vi "GoToTest.vi"(8 "command\nenum":T1, 9 "Robot In":T2={"id"=0, "function"=enum."Attacker", "x"=0.0, "y"=0.0, "orientation"=0.0, "v_tangent"=0.0, "v_normal"=0.0, "v_ang"=0.0, "kick_x"=0.0, "kick_z"=0.0, "dribble"=FALSE, "Timestamp"=timestamp(0 s since 1904-01-01), "dest_x"=0.0, "dest_y"=0.0, "dest_orientation"=0.0, "estimatives"={"est_v_tangent"=0.0, "est_v_normal"=0.0, "est_vx"=0.0, "est_vy"=0.0, "Pos Robot Est"=[]}, "dest_x_kick"=0.0, "dest_y_kick"=0.0, "Gap Coord"=[], "States"=enum."GoToTangent"}, 10 "Ball":dbl[](array[numeric])=[-1986.6092529296875, -3009.6396484375], 11 "GoTo point":dbl[](array[numeric])=[0.0, 0.0, 0.0]) -> (1 "Robot Out":T2={"id"=0, "function"=enum."Attacker", "x"=0.0, "y"=0.0, "orientation"=0.0, "v_tangent"=0.0, "v_normal"=0.0, "v_ang"=0.0, "kick_x"=0.0, "kick_z"=0.0, "dribble"=FALSE, "Timestamp"=timestamp(0 s since 1904-01-01), "dest_x"=0.0, "dest_y"=0.0, "dest_orientation"=0.0, "estimatives"={"est_v_tangent"=0.0, "est_v_normal"=0.0, "est_vx"=0.0, "est_vy"=0.0, "Pos Robot Est"=[]}, "dest_x_kick"=0.0, "dest_y_kick"=0.0, "Gap Coord"=[], "States"=enum."GoToTangent"})   [LabVIEW 2016]
uses:
  Core/AI Robot.ctl
  Intel/Functions Enum.ctl
  Intel/AttackerStates.ctl
  Intel/Command Enum.ctl
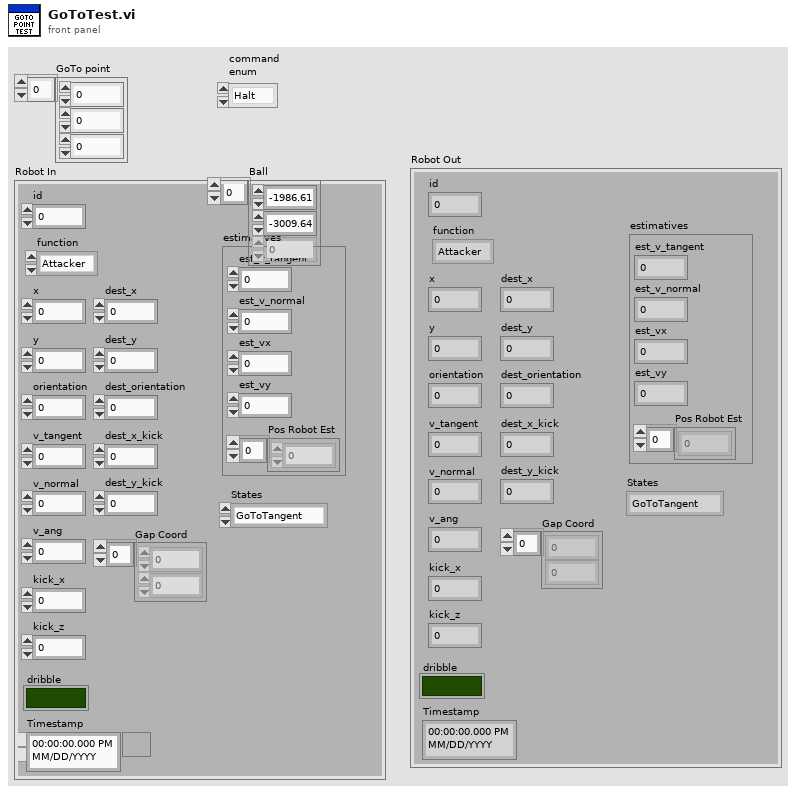
[diagram p1: front panel]
types:
  T1 = typedef "Command Enum.ctl" = enum16{"Halt", "Stop", "Force Start", "PKA Normal Start", "Prepare Kickoff Ally", "PKE Normal Start", "Prepare Kickoff Enemy", "Prepare Penalty Ally", "PPA Normal Start", "Prepare Penalty Enemy", "PPE Normal Start", "Direct Free Enemy", "Direct Free Ally", "Indirect Free Enemy", "Indirect Free Ally", "Timeout Enemy", "Timeout Ally", "Goal Enemy", "Goal Ally", "Ball Placement Enemy", "Ball Placement Ally", "Normal Half Time", "Extra Time Break", "Extra Half Time", "None", "Post Game"}
  T2 = typedef "AI Robot.ctl" = cluster{"id":u32, "function":T3, "x":dbl, "y":dbl, "orientation":dbl, "v_tangent":dbl, "v_normal":dbl, "v_ang":dbl, "kick_x":dbl, "kick_z":dbl, "dribble":bool, "Timestamp":timestamp, "dest_x":dbl, "dest_y":dbl, "dest_orientation":dbl, "estimatives":cluster{"est_v_tangent":dbl, "est_v_normal":dbl, "est_vx":dbl, "est_vy":dbl, "Pos Robot Est":dbl[]}, "dest_x_kick":dbl, "dest_y_kick":dbl, "Gap Coord":dbl[], "States":T4}
  T3 = typedef "Functions Enum.ctl" = enum16{"Attacker", "Goalie", "Defender", "Striker", "Goto 0", "Dummy", "Kicker", "ZigZag"}
  T4 = typedef "AttackerStates.ctl" = enum16{"Pass", "GoToTangent", "BallGetting", "GoToKick", ""}
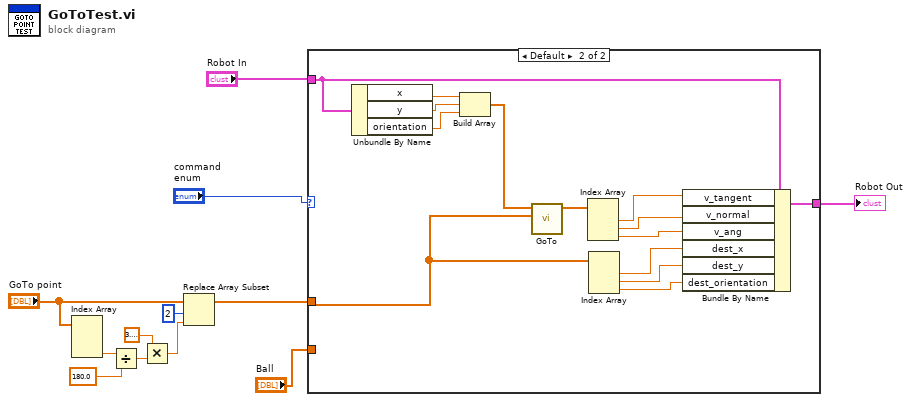
[diagram p0: block diagram]
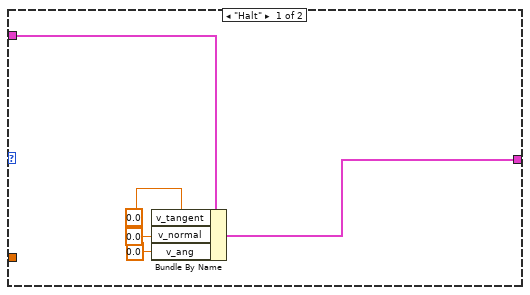
[diagram p2: hidden frame]
diagram:
  n1 = Index Array(array="GoTo point") -> (element #3=w6:dbl)  [unwired: 3 in, 2 out]
  n2 = Divide(x=w6, y=180.0) -> (x/y=w4:dbl)
  n3 = Multiply(x=3.141592653589793, y=w4) -> (x*y=w3:dbl)
  n4 = Replace Array Subset(array="GoTo point", new element=w3, index=2) -> (w7:dbl[])
  n5 = case shown="Default" "command\nenum" {
    tunnel: [w13 w22] -> w11
    tunnel: "Robot In" -> [w17 w27]
    tunnel: w7 -> [_ w19]
    tunnel: "Ball" -> [_ _]
    frame "Halt" {
      n6 = Bundle By Name(cluster=w17, "v_tangent"=0.0, "v_normal"=0.0, "v_ang"=0.0) -> (w13:T2)
    }
    frame Default {
      n7 = Unbundle By Name(w27) -> ("x"=w31:dbl, "y"=w30:dbl, "orientation"=w29:dbl)
      n8 = Build Array(w31, w30, w29) -> (w28:dbl[])
      n9 = call "GoTo.vi"("Target"=w19, "Position"=w28) -> ("Output\nVelocity"=w26:dbl[])  [unwired: 8 in, 1 out]
      n10 = Index Array(array=w26) -> (element #1=w25:dbl, element #2=w24:dbl, element #3=w23:dbl)  [unwired: 3 in]
      n11 = Index Array(array=w19) -> (element #1=w21:dbl, element #2=w20:dbl, element #3=w18:dbl)  [unwired: 3 in]
      n12 = Bundle By Name(cluster=w27, "v_tangent"=w25, "v_normal"=w24, "v_ang"=w23, "dest_x"=w21, "dest_y"=w20, "dest_orientation"=w18) -> (w22:T2)
    }
  }
  "Robot Out" <- w11
